vi "Arm Controller.vi"(8 "error in":errorcluster) -> ()   [LabVIEW 2017]
doc: "This VI executes continuously carrying out the current operation and responding to updates or new operations. It will often contain the timing or control code that is difficult to place directly in TeleOp. This VI generally opens all sensors and motors and isolates the rest of the robot code from knowing how the operations are carried out."
uses:
  <vilib>/Rock Robotics/WPI/Framework/Completion Status.ctl
  Arm Setpoints.ctl
  Arm Operations.ctl
  <vilib>/Rock Robotics/WPI/SafetyOutput/WPI_SafetyOutputConfigMenu.ctl
  <vilib>/Rock Robotics/SystemInterfaces/DIO/FPGA_DIOPWMChannel.ctl
  <vilib>/Rock Robotics/WPI/RobotDrive/WPI_RobotDriveOpen2MotorWithTalonSRX.vi
  <vilib>/Rock Robotics/Network Tables/NT Write Number.vi
panel:
  in  "Interactive Values":T1
  out "Current\nCmd":string
  in  "Buttons":cluster{"Execute Cmd":bool, "Abort Cmd":bool}
  out "Command Timing":cluster{"Start Time (ms)":u32, "Iterations":i32}
  out "Status":T3
  # "Tip: It may be helpful to observe inputs and sensor values.\nYou may also want to display tuning or debugging controls."
  # "Interactive Command: You may fill in the settings for a command\nand schedule it with the Execute button. You can observe and abort\nany command while fine tuning the code for the controller."
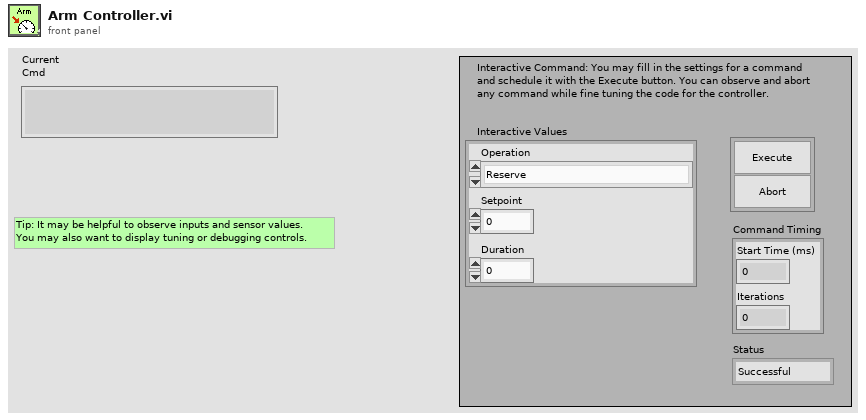
[diagram p1: front panel]
types:
  T1 = typedef "Arm Setpoints.ctl" = cluster{"Operation":T2, "Setpoint":dbl, "Duration":dbl}
  T2 = typedef "Arm Operations.ctl" = enum16{"Reserve", "Read Current", "Immediate", "Move Arm for duration", "Lift Arm", "Lower Arm", "Stop Arm"}
  T3 = typedef "Completion Status.ctl" = enum16{"Successful", "Aborted", "Incomplete"}
  T4 = typedef "FPGA_DIOPWMChannel.ctl" = enum8{"PWM 0", "PWM 1", "PWM 2", "PWM 3", "PWM 4", "PWM 5", "PWM 6", "PWM 7", "PWM 8", "PWM 9", "PWM MXP 0", "PWM MXP 1", "PWM MXP 2", "PWM MXP 3", "PWM MXP 4", "PWM MXP 5", "PWM MXP 6", "PWM MXP 7", "PWM MXP 8", "PWM MXP 9", "Invalid"}
  T5 = typedef "WPI_SafetyOutputConfigMenu.ctl" = enum16{"Enable", "Disable"}
  T6 = typedef "WPI_RobotDriveDevRef.ctl" = cluster{"DevStatus":errorcluster, "Motors[]":T7[], "Square Inputs":bool, "Max Output":dbl}
  T7 = typedef "WPI_MotorControlDeviceRef.ctl" = cluster{"DeviceStatus":errorcluster, "Type":T8, "PWM":cluster{"PWM Channel":T4, "DeadBand":T9}, "CAN":cluster{"Device Number":u8, "SetOutput VI Ref":variant, "GetOutput VI Ref":variant, "Enable VI Ref":variant, "Disable VI Ref":variant, "Data":variant}, "Invert":bool, "DIO PWM":cluster{"PWM \"Enable\" Channel":T4, "DIOChannel":T10, "PWM Rate":dbl}}
  T8 = typedef "WPI_MotorControlType.ctl" = enum16{"PWM", "CAN", "DIO PWM"}
  T9 = typedef "WPI_PWMDeadband.ctl" = cluster{"Name":string, "maxPositivePwm":i32, "minPositivePwm":i32, "centerPwm":i32, "maxNegativePwm":i32, "minNegativePwm":i32, "angularRange":u16}
  T10 = typedef "FPGA_DIOChannel.ctl" = enum8{"DIO 0", "DIO 1", "DIO 2", "DIO 3", "DIO 4", "DIO 5", "DIO 6", "DIO 7", "DIO 8", "DIO 9", "DIO MXP 0", "DIO MXP 1", "DIO MXP 2", "DIO MXP 3", "DIO MXP 4", "DIO MXP 5", "DIO MXP 6", "DIO MXP 7", "DIO MXP 8", "DIO MXP 9", "DIO MXP 10", "DIO MXP 11", "DIO MXP 12", "DIO MXP 13", "DIO MXP 14", "DIO MXP 15", "SPI Port CS1", "SPI Port CS2", "SPI Port CS3", "SPI Port MISO", "SPI Port MOSI", "Invalid"}
  T11 = typedef "Command Status Info.ctl" = cluster{"Name":string, "Status":T3, "notifier out":T12}
  T12 = typedef "Completion Notifier.ctl" = refnum<notifier>
  T13 = cluster{"Current Command":T1, "Command Timing":cluster{"Start Time (ms)":u32, "Iterations":i32}, "Command Arguments":cluster{"Command Info":T11, "Description":string, "Default Command":T1, "queue out":refnum<queue>, "Subsystem Name":string}}
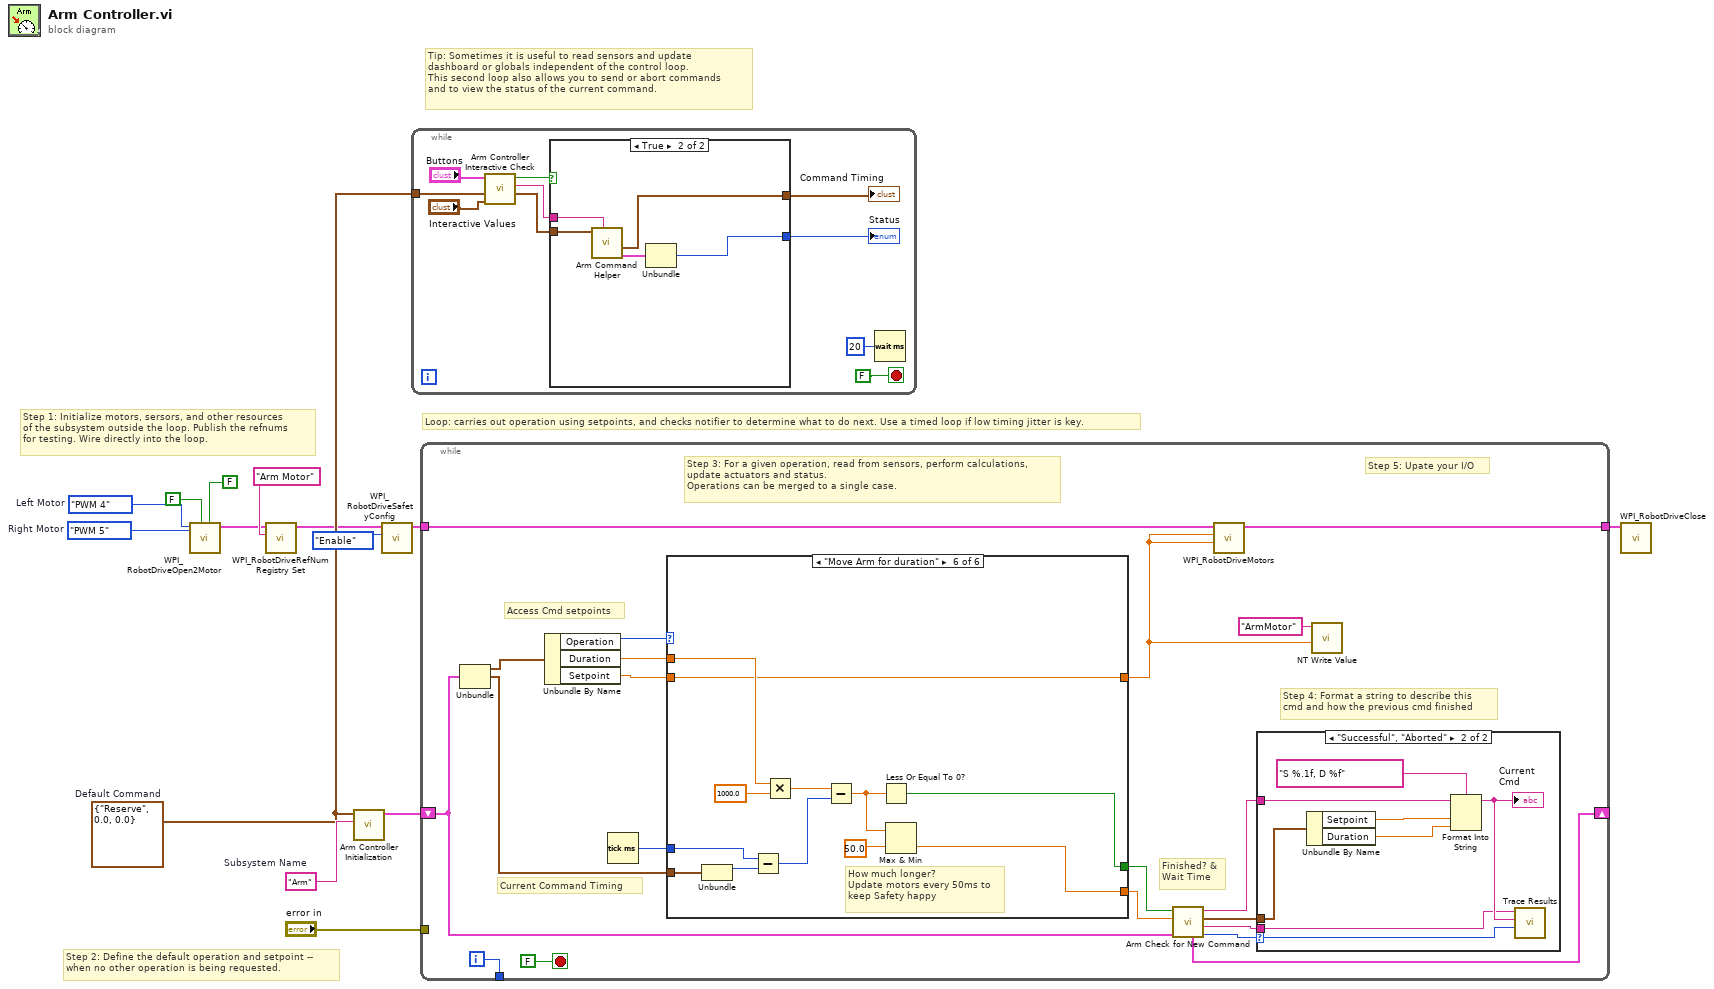
[diagram p0: block diagram]
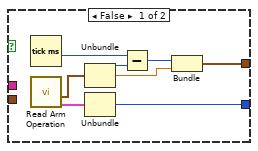
[diagram p2: hidden frame]
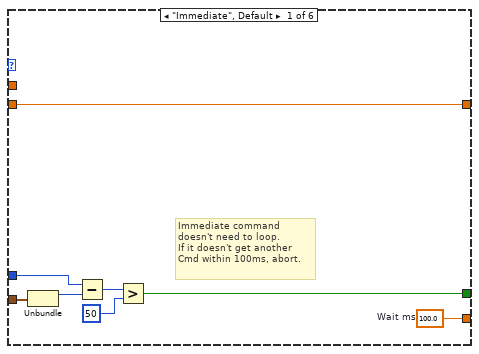
[diagram p4: hidden frame]
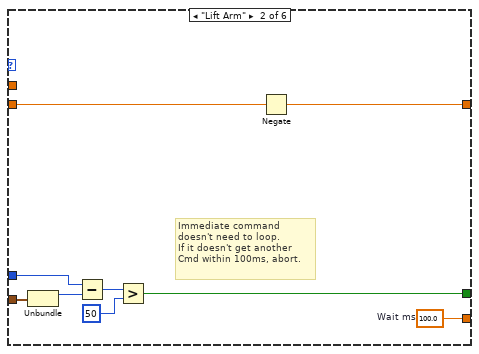
[diagram p5: hidden frame]
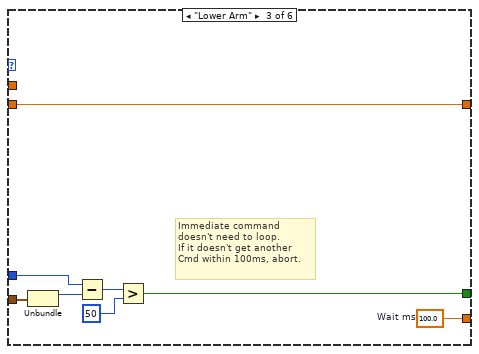
[diagram p6: hidden frame]
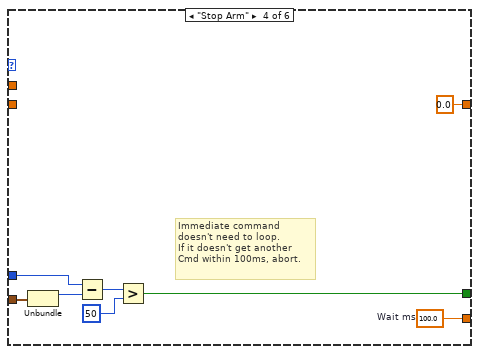
[diagram p7: hidden frame]
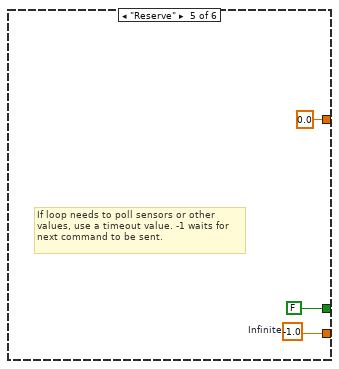
[diagram p8: hidden frame]
diagram:
  w4 = FPGA_DIOPWMChannel."PWM 5"  # Right Motor
  w1 = FPGA_DIOPWMChannel."PWM 4"  # Left Motor
  w11 = T1 {"Operation"=enum."Reserve", "Setpoint"=0.0, "Duration"=0.0}  # Default Command
  w12 = "Arm"  # Subsystem Name
  # "Tip: Sometimes it is useful to read sensors and update\ndashboard or globals independent of the control loop.\nThis second loop also allows you to send or abort commands\nand to view the status of the current command."
  # "Step 2: Define the default operation and setpoint --\nwhen no other operation is being requested."
  # "Step 1: Initialize motors, sersors, and other resources\nof the subsystem outside the loop. Publish the refnums\nfor testing. Wire directly into the loop."
  # "Loop: carries out operation using setpoints, and checks notifier to determine what to do next. Use a timed loop if low timing jitter is key."
  n1 = call-poly <vilib>:"WPI_RobotDriveOpen2Motor.vi"("Right Motor Inverted"=FALSE, "Left Motor Inverted"=FALSE, "Right Motor"=w4, "Left Motor"=w1) -> ("RobotDriveDevRef"=w7:T6)  [unwired: 6 in, 1 out]
  n2 = call <vilib>:"WPI_RobotDriveRefNum Registry Set.vi"("refnum name"="Arm Motor", "RobotDriveDevRef"=w7) -> ("RobotDriveDevRef"=w6:T6)  [unwired: 8 in, 1 out]
  n3 = call "Arm Controller Initialization.vi"("Subsystem Name"=w12, "Default Command"=w11) -> ("Current Command"=w13:T13)  [unwired: 9 in]
  n4 = call <vilib>:"WPI_RobotDriveSafetyConfig.vi"("mode"=WPI_SafetyOutputConfigMenu."Enable", "RobotDriveDevRef"=w6) -> ("RobotDriveDevRef"=w8:T6)  [unwired: 8 in, 1 out]
  n5 = while {
    tunnel: w11 -> [w21]
    stop <- FALSE stop-if-true
    n6 = call "Arm Controller Interactive Check.vi"("Interactive Command in"="Interactive Values", "Default Command"=w21, "Buttons"="Buttons") -> ("Interactive Command out"=w18:T1, "Trace String"=w19:string, "Schedule"=w20:bool)  [unwired: 6 in]
    n7 = case shown="True" w20 {
      tunnel: [w32 w37] -> w17
      tunnel: w18 -> [_ w35]
      tunnel: [w28 w33] -> w16
      tunnel: w19 -> [_ w36]
      frame False {
        n8 = Tick Count (ms)() -> (millisecond timer value=w27:u32)
        n9 = call "Read Arm Operation.vi"() -> ("Command Info"=w25:T11, "SubSystem Data"=w26:T1)  [unwired: 9 in, 1 out]
        n10 = Unbundle(w26) -> ("Operation"=w31:T2, "Setpoint"=w29:dbl)  [unwired: 1 out]
        n11 = Unbundle(w25) -> ("Status"=w32:T3)  [unwired: 2 out]
        n12 = Subtract(x=w27, y=w31) -> (x-y=w30:u32)
        n13 = Bundle(w30, "Setpoint"=w29) -> (w28:cluster{u32, "Setpoint":dbl})  [unwired: 1 in]
      }
      frame True {
        n14 = call "Arm Command Helper.vi"("Description"=w36, "SubSystem Data"=w35) -> ("Command Info Out"=w34:T11, "Command Timing"=w33:cluster{"Start Time (ms)":u32, "Iterations":i32})  [unwired: 7 in, 1 out]
        n15 = Unbundle(w34) -> ("Status"=w37:T3)  [unwired: 2 out]
      }
    }
    "Status" <- w17
    "Command Timing" <- w16
    n16 = Wait (ms)(milliseconds to wait=u32 20) -> ()  [unwired: 1 out]
  }
  n17 = while {
    shift-right: [w49] -> _
    shift-left: w13 -> [w42]
    tunnel: [w56] -> _
    tunnel: "error in" -> [_]
    tunnel: w8 -> [w39]
    tunnel: [w41] -> w5
    i -> [w56]
    stop <- FALSE stop-if-true
    # "Step 5: Upate your I/O"
    # "Step 4: Format a string to describe this\ncmd and how the previous cmd finished"
    # "Current Command Timing"
    # "Access Cmd setpoints"
    # "Finished? &\nWait Time"
    # "Step 3: For a given operation, read from sensors, perform calculations,\nupdate actuators and status.\nOperations can be merged to a single case."
    n18 = Unbundle(w42) -> ("Current Command"=w55:T1, "Command Timing"=w51:cluster{"Start Time (ms)":u32, "Iterations":i32})  [unwired: 1 out]
    n19 = Unbundle By Name(w55) -> ("Operation"=w54:T2, "Duration"=w53:dbl, "Setpoint"=w50:dbl)
    n20 = Tick Count (ms)() -> (millisecond timer value=w52:u32)
    n21 = case shown="\"Move Arm for duration\"" w54 {
      tunnel: [w73 w82 w90 w98 w101 w103] -> w47
      tunnel: [w67 w76 w84 w92 FALSE ("ignore previous (F)") w104] -> w48
      tunnel: w51 -> [w69 w78 w86 w94 _ w107]
      tunnel: w53 -> [_ _ _ _ _ w105]
      tunnel: w52 -> [w68 w77 w85 w93 _ w106]
      tunnel: w50 -> [w66 w75 w83 _ _ w102]
      tunnel: [w66 w74 w83 0.0 ("Setpoint") 0.0 ("Setpoint") w102] -> w38
      frame "Immediate", Default {
        w73 = 100.0  # Wait ms
        # "Immediate command\ndoesn't need to loop.\nIf it doesn't get another\nCmd within 100ms, abort."
        n22 = Unbundle(w69) -> ("Start Time (ms)"=w72:u32)  [unwired: 1 out]
        n23 = Subtract(x=w68, y=w72) -> (x-y=w71:u32)
        n24 = Greater?(x=w71, y=u8 50 ("Left Motor")) -> (0:w67:bool)
      }
      frame "Lift Arm" {
        w82 = 100.0  # Wait ms
        # "Immediate command\ndoesn't need to loop.\nIf it doesn't get another\nCmd within 100ms, abort."
        n25 = Unbundle(w78) -> ("Start Time (ms)"=w81:u32)  [unwired: 1 out]
        n26 = Subtract(x=w77, y=w81) -> (x-y=w80:u32)
        n27 = Greater?(x=w80, y=u8 50 ("Left Motor")) -> (0:w76:bool)
        n28 = Negate(x=w75) -> (-x=w74:dbl)
      }
      frame "Lower Arm" {
        w90 = 100.0  # Wait ms
        # "Immediate command\ndoesn't need to loop.\nIf it doesn't get another\nCmd within 100ms, abort."
        n29 = Unbundle(w86) -> ("Start Time (ms)"=w89:u32)  [unwired: 1 out]
        n30 = Subtract(x=w85, y=w89) -> (x-y=w88:u32)
        n31 = Greater?(x=w88, y=u8 50 ("Left Motor")) -> (0:w84:bool)
      }
      frame "Stop Arm" {
        w98 = 100.0  # Wait ms
        # "Immediate command\ndoesn't need to loop.\nIf it doesn't get another\nCmd within 100ms, abort."
        n32 = Unbundle(w94) -> ("Start Time (ms)"=w97:u32)  [unwired: 1 out]
        n33 = Subtract(x=w93, y=w97) -> (x-y=w96:u32)
        n34 = Greater?(x=w96, y=u8 50 ("Left Motor")) -> (0:w92:bool)
      }
      frame "Reserve" {
        w101 = -1.0  # Infinite
        # "If loop needs to poll sensors or other\nvalues, use a timeout value. -1 waits for\nnext command to be sent."
      }
      frame "Move Arm for duration" {
        # "How much longer?\nUpdate motors every 50ms to\nkeep Safety happy"
        n35 = Unbundle(w107) -> ("Start Time (ms)"=w110:u32)  [unwired: 1 out]
        n36 = Subtract(x=w106, y=w110) -> (x-y=w113:u32)
        n37 = Multiply(x=w105, y=1000.0) -> (x*y=w112:dbl)
        n38 = Subtract(x=w112, y=w113) -> (x-y=w109:dbl)
        n39 = Less Or Equal To 0?(x=w109) -> (x <= 0?=w104:bool)
        n40 = Max & Min(x=w109, y=50.0) -> (min(x,y)=w103:dbl)  [unwired: 1 out]
      }
    }
    n41 = call "Arm Check for New Command.vi"("Current Command"=w42, "Wait time (ms)"=w47, "Finished?"=w48) -> ("Completion"=w43:T3, "Subsystem Name"=w44:string, "Current Command"=w45:T1, "Initial Trace String"=w46:string, "NextCommand"=w49:T13)  [unwired: 4 in]
    n42 = call <vilib>:"WPI_RobotDriveMotors.vi"("RightSpeed"=w38, "LeftSpeed"=w38, "RobotDriveDevRef"=w39) -> ("RobotDriveDevRef"=w41:T6)  [unwired: 6 in, 2 out]
    n43 = case shown="\"Successful\", \"Aborted\"" w43 {
      selector: w43 -> [_ w65]
      tunnel: w46 -> [_ w61]
      tunnel: w45 -> [_ w62]
      tunnel: w44 -> [_ w58]
      frame "Incomplete", Default {
        # "Continuing current command"
      }
      frame "Successful", "Aborted" {
        # "Report and setup for next command"
        n44 = Unbundle By Name(w62) -> ("Setpoint"=w64:dbl, "Duration"=w59:dbl)
        n45 = Format Into String(format string="S %.1f, D %f", initial string=w61, w64, w59) -> (resulting string=w60:string)  [unwired: 1 in, 1 out]
        "Current\nCmd" <- w60
        n46 = call <vilib>:"Trace Results.vi"("Status of previous command"=w65, "Description"=w60, "Subsystem"=w58) -> ()  [unwired: 9 in]
      }
    }
    n47 = call-poly <vilib>:"NT Write Value.vi"("Numeric"=w38, "Name"="ArmMotor") -> ()  [unwired: 9 in, 1 out]
  }
  n48 = call <vilib>:"WPI_RobotDriveClose.vi"("RobotDriveDevRef"=w5) -> ()  [unwired: 10 in, 1 out]
